vi "Actor Core.vi"(8 "error in":errorcluster, 11 "Nested":refnum<class "Nested.lvclass">) -> (0 "error out":errorcluster, 3 "Actor out":refnum<class "Actor.lvclass">)   [LabVIEW 2019, in "Nested.lvlib" / "Nested.lvclass"]
doc: "(<B>Filename</B>: Actor Framework.lvlib:Actor.lvclass:Actor Core.vi)\n\nReceives messages to the actor, reacts to them, and initiates any error handling that may shut the actor down.\n\nDescendant classes may override this VI to append parallel tasks for the actor to complete while it handles messages. Overrides use the Call Parent Class Method node."
uses:
  Nested.lvclass
  C:/Program Files (x86)/National Instruments/LabVIEW 2019/vi.lib/ActorFramework/Actor/Actor.lvclass
  <vilib>/ActorFramework/Actor/Actor.lvclass
  <vilib>/ActorFramework/Actor/Actor.lvclass/Actor.ctl
  <vilib>/ActorFramework/Message Enqueuer/Message Enqueuer.lvclass/Message Enqueuer.ctl
  <vilib>/ActorFramework/Message Enqueuer/Init from Existing Queue.vi
  <vilib>/ActorFramework/Message Enqueuer/Enqueue.vi
  <vilib>/ActorFramework/Stop Msg/Stop Msg.lvclass
  C:/Program Files (x86)/National Instruments/LabVIEW 2019/vi.lib/ActorFramework/Message/Message.lvclass
  <vilib>/ActorFramework/Message Priority Queue/Priority Enqueue.vi
  <vilib>/ActorFramework/Message Enqueuer/Message Enqueuer.lvclass
panel:
  in  "Stop Window":bool
  in  "Reset":bool
  out "Counter":i32
  in  "Wait (ms)":i32=500
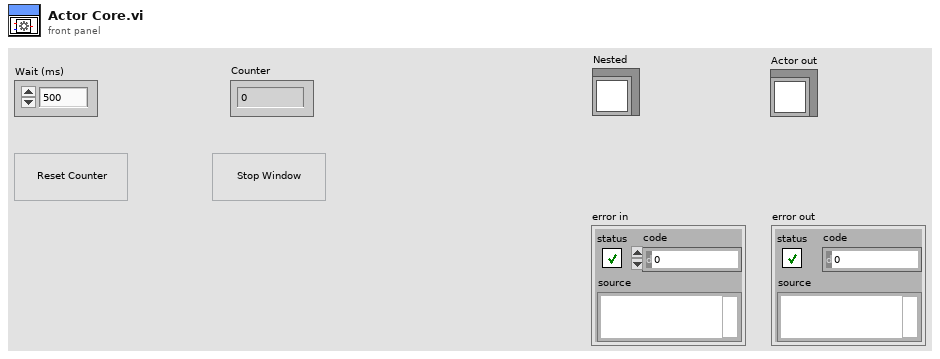
[diagram p1: front panel]
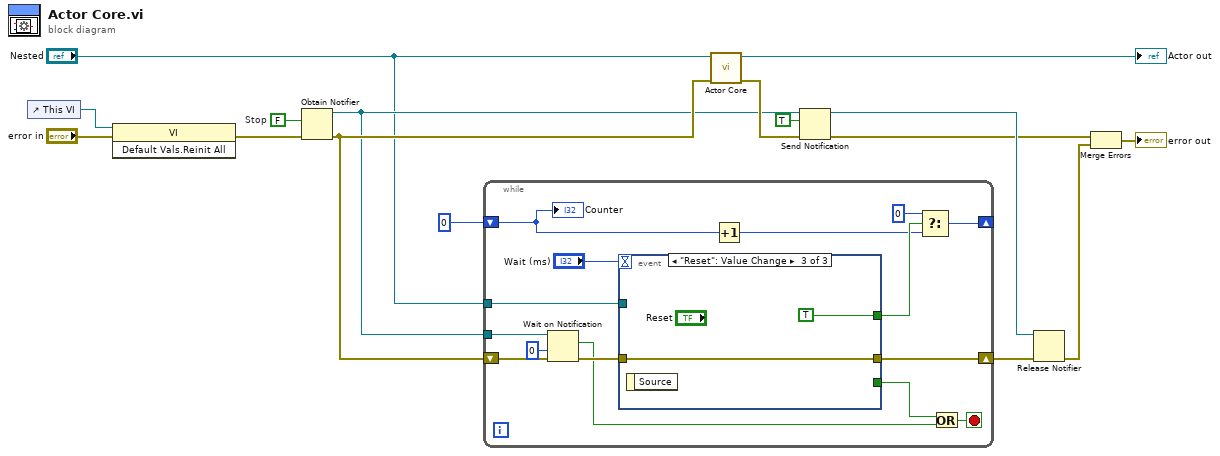
[diagram p0: block diagram]
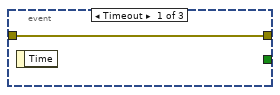
[diagram p2: hidden frame]
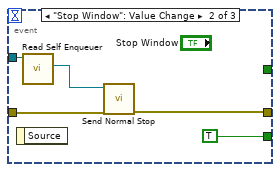
[diagram p3: hidden frame]
diagram:
  w2 = FALSE  # Stop
  n1 = control-ref of="This VI"() -> (w4:refnum<vi>)
  n2 = invoke class="VI" method="Default Vals.Reinit All"(reference=w4, error in="error in") -> (error out=w3:errorcluster)  [unwired: 1 in, 2 out]
  n3 = Obtain Notifier(notification data type=w2, error in (no error)=w3) -> (notifier out=w12:refnum<notifier>, error out=w13:errorcluster)  [unwired: 2 in, 1 out]
  n4 = while {
    tunnel: w12 -> [w30]
    shift-right: [w23] -> w11
    shift-left: w13 -> [w31]
    tunnel: "Nested" -> [w22]
    shift-right: [w20] -> _
    shift-left: 0 -> [w21]
    stop <- w26 stop-if-true
    n5 = Wait on Notification(notifier=w30, timeout in ms (-1)=0, error in (no error)=w31) -> (notification=w25:bool, error out=w28:errorcluster)  [unwired: 1 in, 2 out]
    n6 = event shown="[2] \"Reset\": Value Change" {
      selector: _ -> [_ _ _]
      dyn-events: _ -> [_ _ _]
      timeout: "Wait (ms)" -> [_ _ _]
      tunnel: w28 -> [w32 w35 w38]
      tunnel: [_ TRUE ("x") _] -> w24
      tunnel: [w32 w33 w38] -> w23
      tunnel: w22 -> [_ w36 _]
      tunnel: [_ _ TRUE ("x")] -> w19
      event Timeout {
        n7 = event-data() -> ()  [unwired: 1 in, 1 out]
      }
      event "Stop Window": Value Change {
        n8 = event-data() -> ()  [unwired: 1 in, 1 out]
        n9 = call <vilib>:"Read Self Enqueuer.vi"("Actor"=w36) -> ("Self Enqueuer"=w34:refnum<class "Message Enqueuer.lvclass">)  [unwired: 10 in]
        n10 = call <vilib>:"Send Normal Stop.vi"("error in (no error)"=w35, "Message Enqueuer"=w34) -> ("error out"=w33:errorcluster)  [unwired: 9 in]
      }
      event "Reset": Value Change {
        n11 = event-data() -> ()  [unwired: 1 in, 1 out]
      }
    }
    n12 = Increment(x=w21) -> (x+1=w17:i32)
    n13 = Select(t=0, s=w19, f=w17) -> (s? t:f=w20:i32)
    n14 = Or(x=w24, y=w25) -> (x .or. y?=w26:bool)
    "Counter" <- w21
  }
  n15 = call-parent "Actor Core.vi"("error in"=w13, "Actor in"="Nested") -> ("error out"=w15:errorcluster, "Actor out"=→"Actor out":refnum<class "Actor.lvclass">)  [unwired: 8 in]
  n16 = Send Notification(notification=TRUE, notifier=w12, error in (no error)=w15) -> (notifier out=w10:refnum<notifier>, error out=w9:errorcluster)
  n17 = Release Notifier(notifier=w10, error in (no error)=w11) -> (error out=w7:errorcluster)  [unwired: 1 in, 2 out]
  n18 = Merge Errors(w9, w7) -> (→"error out":errorcluster)
